vi "Driving Controller Vi.vi"(8 "Obs Distances Measure Array":dbl[](array[numeric]), 9 "Posture In":dbl[](array[numeric]), 10 "Goal Frame (World)":cluster{"X":sgl, "Y":sgl, "Theta":dbl}, 11 "Robot Frame (World)":cluster{"X":sgl, "Y":sgl, "Theta":dbl}) -> (2 "Goal Arrived?":bool, 3 "Frame Velocity":dbl[](array[numeric]))   [LabVIEW 2016]
uses:
  RunningState.ctl
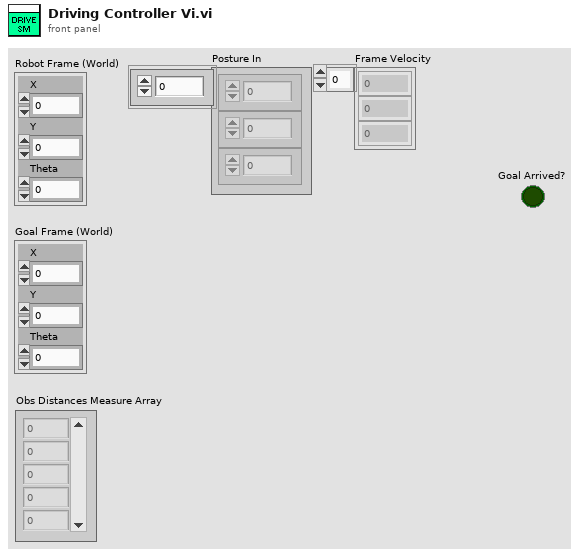
[diagram p1: front panel]
types:
  T1 = typedef "RunningState.ctl" = enum16{"GTG and AO", "Go To Goal", "Wait", "Next Goal", "Avoid Obstacle", "Stop at Goal"}
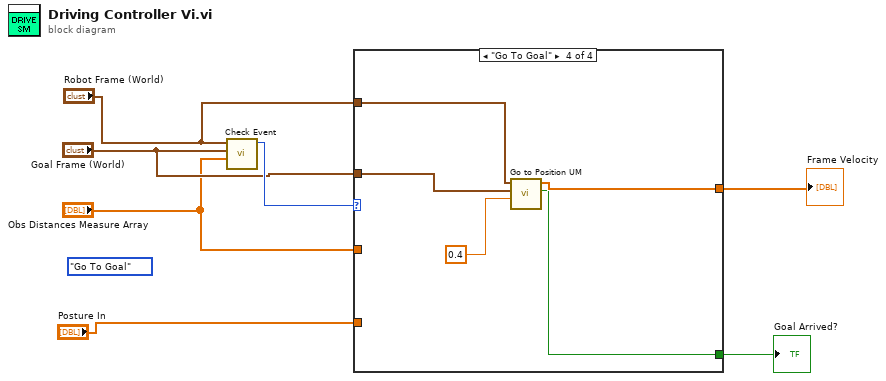
[diagram p0: block diagram]
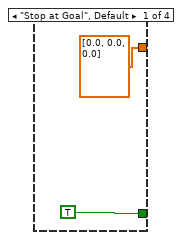
[diagram p2: hidden frame]
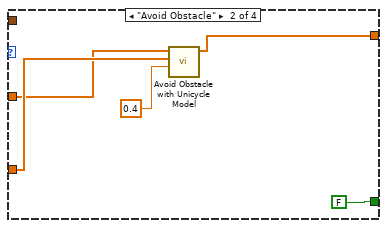
[diagram p3: hidden frame]
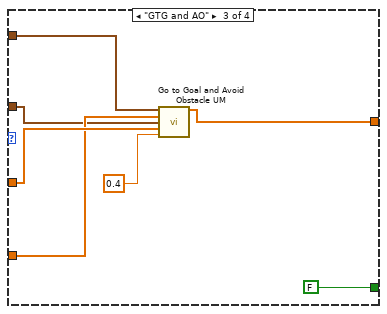
[diagram p4: hidden frame]
diagram:
  (unwired) RunningState."Go To Goal" ("Enum")
  n1 = call "Check Event.vi"("Distances Measure Array"="Obs Distances Measure Array", "Goal Frame (World)"="Goal Frame (World)", "Robot Frame (World)"="Robot Frame (World)") -> ("Current Event"=w6:T1)  [unwired: 8 in]
  n2 = case shown="\"Go To Goal\"" w6 {
    tunnel: [TRUE FALSE FALSE w22] -> w7
    tunnel: "Robot Frame (World)" -> [_ _ w20 w26]
    tunnel: "Goal Frame (World)" -> [_ _ w15 w25]
    tunnel: [dbl[] [0.0, 0.0, 0.0] ("Frame Velocity") w11 w17 w23] -> w3
    tunnel: "Obs Distances Measure Array" -> [_ w12 w19 _]
    tunnel: "Posture In" -> [_ w13 w16 _]
    frame "Stop at Goal", Default {
    }
    frame "Avoid Obstacle" {
      n3 = call "Avoid Obstacle with Unicycle Model.vi"("V forward"=0.4, "Posture In"=w13, "IF readings\n(meters)"=w12) -> ("Frame Velocity"=w11:dbl[])  [unwired: 8 in]
    }
    frame "GTG and AO" {
      n4 = call "Go to Goal and Avoid Obstacle UM.vi"("Robot Frame (World)"=w20, "Posture In"=w16, "Goal Frame (World)"=w15, "IF readings\n(meters)"=w19, "V Forward"=0.4) -> ("Frame Velocity"=w17:dbl[])  [unwired: 10 in]
    }
    frame "Go To Goal" {
      n5 = call "Go to Position UM.vi"("V Forward"=0.4, "Goal Frame (World)"=w25, "Robot Frame (World)"=w26) -> ("Arrive?"=w22:bool, "Frame Velocity"=w23:dbl[])  [unwired: 5 in]
    }
  }
  "Goal Arrived?" <- w7
  "Frame Velocity" <- w3
